vi "Launcher.vi"() -> ()   [LabVIEW 2021, in "Secure Echo Broadcast Test With Server Manager.lvlib"]
uses:
  Secure Echo Broadcast Test With Server Manager.lvlib
  WebSocket Actor/WebSocket Connection/Keepalive.ctl
  WS Test Server Subscriber/WS Test Server Subscriber.lvclass
  C:/Program Files/National Instruments/LabVIEW 2021/vi.lib/ActorFramework/Actor/Actor.lvclass
  WebSocket Actor/WebSocket Server Manager/WebSocket Server Manager.lvclass
  WebSocket Actor/WebSocket Server Manager/WebSocket Server Manager.lvclass/WebSocket Server Manager.ctl
  WS Test Server Subscriber/WS Test Server Subscriber.lvclass/WS Test Server Subscriber.ctl
  WS Test Client Subscriber/WS Test Client Subscriber.lvclass
  WS Test Client Subscriber/WS Test Client Subscriber.lvclass/WS Test Client Subscriber.ctl
  <vilib>/ActorFramework/Message Enqueuer/Message Enqueuer.lvclass/Message Enqueuer.ctl
  WS Test Client Subscriber/Write Keepalive.vi
  WS Test Client Subscriber/Write Certificate.vi
  WebSocket Actor/WebSocket Server Manager/Write Keepalive.vi
  WebSocket Actor/WebSocket Server Manager/Write Certificate Chain.vi
  WebSocket Actor/WebSocket Server Manager/Write Private Key.vi
  WebSocket Actor/WebSocket Server Manager/Write Secure.vi
  WS Test Server Subscriber/properties/Write WebSocket Server Manager Enqueuer.vi
  <vilib>/ActorFramework/Message Enqueuer/Enqueue.vi
  <vilib>/ActorFramework/Stop Msg/Stop Msg.lvclass
  C:/Program Files/National Instruments/LabVIEW 2021/vi.lib/ActorFramework/Message/Message.lvclass
  <vilib>/Utility/LVClass/Get LV Class Name.vi
  <resource>/AFDebug/Generate Trace for Message.vi
  <vilib>/ActorFramework/Message Priority Queue/Priority Enqueue.vi
  <vilib>/ActorFramework/Actor/Actor.lvclass
  <userlib>/_OpenG.lib/time/time.llb/openg_time.lvlib
  WebSocket Actor/WebSocket Connection/WebSocket Connection.lvclass
panel:
  in  "Keepalive":T1={"Enabled"=TRUE, "Ping Interval (ms)"=25000, "Ping Timeout (ms)"=20000}
  in  "Stop Actors":bool
  in  "Number of Clients":i32=3
  out "error out":errorcluster
  # "In this example we will use the Server Manager Actor Infrastructure to launch a Secure WebSocket Server and we will illustrate a secure bidirectional communication between the WebSocket server and clients. \nWe launch one server that will define the /echo/ service. Then a user selectable number of clients can be launched. From such clients messages to the servers can be sent on the specified service. The server will echo back the message to the clients. The server can broadcast messages to the clients. One can choose to send a series of messages at a certain time frequency. \n\nInstructions to execute the example:\n1. open with Administrator rights the following file \"C:\\Windows\\System32\\drivers\\etc\\hosts\"\n2. add as new line the following text \"127.0.0.1       lvtls.example\" without quotes\n3. Reboot your PC\n4. Run this VI\n5. Wait that the Server and Client GUI appear\n6. use the GUIs to exchange messages\n7. Stop the actors from this VI"
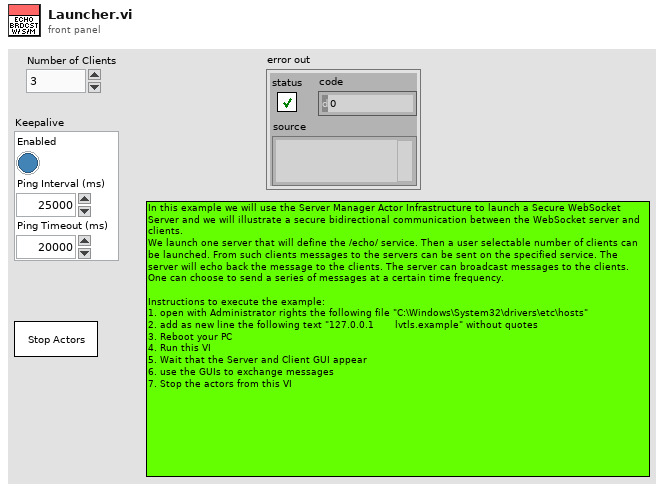
[diagram p1: front panel]
types:
  T1 = typedef "WebSocket Actors.lvlib/WebSocket Connection.lvclass/Keepalive.ctl" = cluster{"Enabled":bool, "Ping Interval (ms)":u32, "Ping Timeout (ms)":u32}
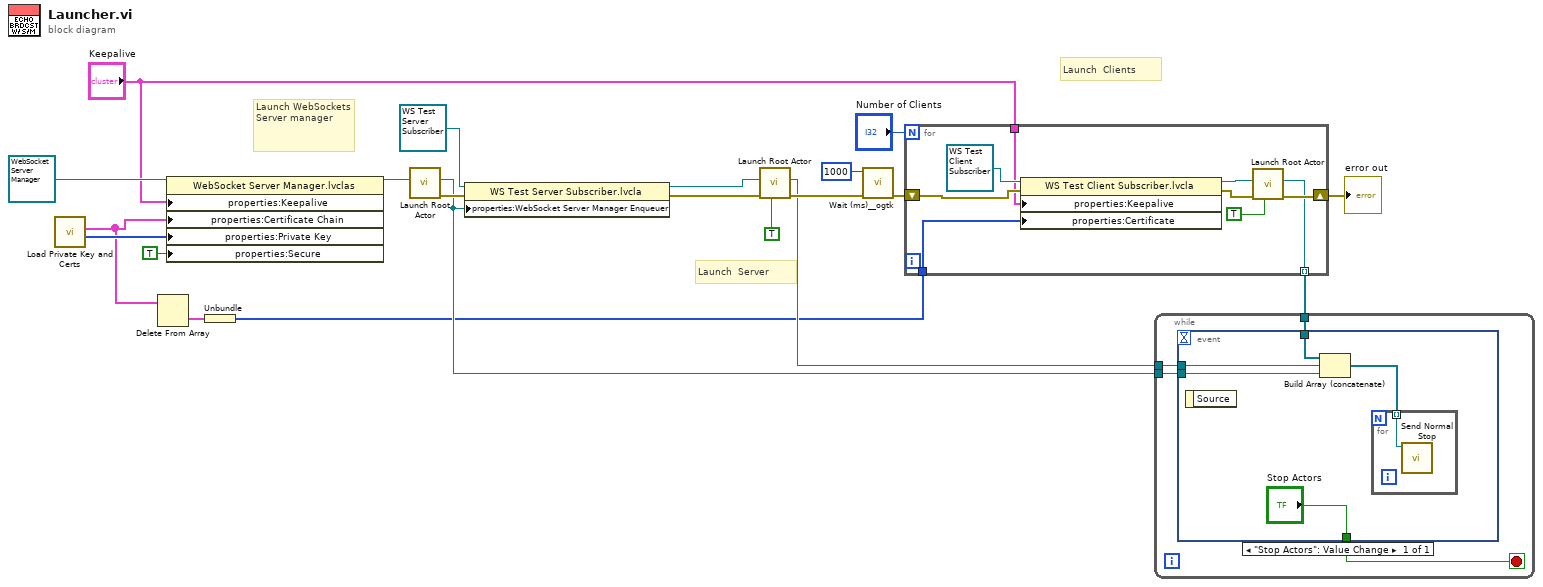
[diagram p0: block diagram]
diagram:
  # "Launch  Clients"
  # "Launch  Server"
  # "Launch WebSockets Server manager"
  n1 = call "Load Private Key and Certs.vi"() -> ("Private Key"=w5:u8[], "Certificate Chain"=w2:cluster{"certificate":u8[]}[])  [unwired: 9 in, 1 out]
  n2 = Delete From Array(array=w2) -> (deleted portion=w3:cluster{"certificate":u8[]})  [unwired: 2 in, 1 out]
  n3 = property class="WebSocket Server Manager.lvclas"(reference=refnum<class "WebSocket Server Manager.lvclass"> refnum ("WebSocket Actors.lvlib:WebSocket Server Manager.lvclass"), "properties:Keepalive"="Keepalive", "properties:Certificate Chain"=w2, "properties:Private Key"=w5, "properties:Secure"=TRUE ("Secure")) -> (reference out=w7:refnum<class "WebSocket Server Manager.lvclass">)  [unwired: 1 in, 1 out]
  n4 = Unbundle(w3) -> ("certificate"=w1:u8[])
  n5 = call <vilib>:"Launch Root Actor.vi"("Actor"=w7) -> ("error out"=w15:errorcluster, "Actor's Enqueuer"=w11:refnum<class "Message Enqueuer.lvclass">)  [unwired: 9 in]
  n6 = property class="WS Test Server Subscriber.lvcla"(reference=refnum<class "WS Test Server Subscriber.lvclass"> refnum ("WS Full LabVIEW Test.lvlib:WS Test Server.lvclass"), error in=w15, "properties:WebSocket Server Manager Enqueuer"=w11) -> (reference out=w16:refnum<class "WS Test Server Subscriber.lvclass">, error out=w9:errorcluster)
  n7 = call <vilib>:"Launch Root Actor.vi"("Open Actor Core front panel? (F)"=TRUE, "error in (no error)"=w9, "Actor"=w16) -> ("error out"=w19:errorcluster, "Actor's Enqueuer"=w10:refnum<class "Message Enqueuer.lvclass">)  [unwired: 7 in]
  n8 = call <userlib>:"Wait (ms)__ogtk.vi"("error in (no error)"=w19, "milliseconds to wait"=u32 1000) -> ("error out"=w14:errorcluster)  [unwired: 8 in, 1 out]
  n9 = for {
    N: "Number of Clients" -> [_]
    shift-right: [w28] -> w18
    shift-left: w14 -> [w25]
    tunnel: [w27] -> w8 mode=indexing
    tunnel: "Keepalive" -> [w23]
    tunnel: w1 -> [w22]
    n10 = property class="WS Test Client Subscriber.lvcla"(reference=refnum<class "WS Test Client Subscriber.lvclass"> refnum ("WS Full LabVIEW Test.lvlib:WS Test Client.lvclass"), error in=w25, "properties:Keepalive"=w23, "properties:Certificate"=w22) -> (reference out=w26:refnum<class "WS Test Client Subscriber.lvclass">, error out=w24:errorcluster)
    n11 = call <vilib>:"Launch Root Actor.vi"("Open Actor Core front panel? (F)"=TRUE, "error in (no error)"=w24, "Actor"=w26) -> ("error out"=w28:errorcluster, "Actor's Enqueuer"=w27:refnum<class "Message Enqueuer.lvclass">)  [unwired: 7 in]
  }
  "error out" <- w18
  n12 = while {
    tunnel: w11 -> [w34]
    tunnel: w10 -> [w32]
    tunnel: w8 -> [w31]
    stop <- w33 stop-if-true
    n13 = event shown="[0] \"Stop Actors\": Value Change" {
      selector: _ -> [_]
      dyn-events: _ -> [_]
      timeout: _ -> [_]
      tunnel: w34 -> [w39]
      tunnel: ["Stop Actors"] -> w33
      tunnel: w32 -> [w36]
      tunnel: w31 -> [w35]
      event "Stop Actors": Value Change {
        n14 = event-data() -> ()  [unwired: 1 in, 1 out]
        n15 = Build Array (concatenate)(w35, w36, w39) -> (w37:refnum<class "Message Enqueuer.lvclass">[])
        n16 = for {
          tunnel: w37 -> [w40] mode=indexing
          n17 = call <vilib>:"Send Normal Stop.vi"("Message Enqueuer"=w40) -> ()  [unwired: 10 in, 1 out]
        }
      }
    }
  }
